vi "Get State from Child.vi"(8 "error in (no error)":errorcluster, 10 "Boolean":bool, 11 "Parent Actor in":refnum<class "Parent Actor.lvclass">) -> (0 "error out":errorcluster, 3 "Parent Actor out":refnum<class "Parent Actor.lvclass">)   [LabVIEW 2012, in "Parent Actor.lvclass"]
uses:
  Parent Actor.lvclass
  Parent Actor.lvclass/Parent Actor.ctl
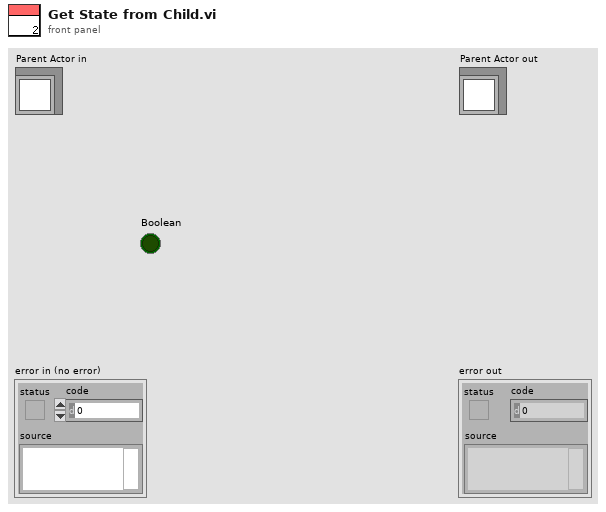
[diagram p1: front panel]
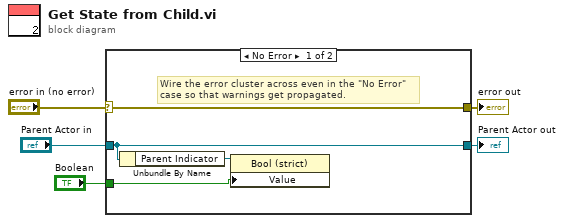
[diagram p0: block diagram]
diagram:
  n1 = case shown="No Error" "error in (no error)" {
    selector: "error in (no error)" -> [w9 w11]
    tunnel: [w9 w11] -> w4
    tunnel: [w8 w10] -> w2
    tunnel: "Parent Actor in" -> [w8 w10]
    tunnel: "Boolean" -> [w6 _]
    frame No Error {
      # "Wire the error cluster across even in the \"No Error\"\ncase so that warnings get propagated."
      n2 = Unbundle By Name(w8) -> ("Parent Indicator"=w7:refnum<vi>)
      n3 = property class="Bool (strict)"(reference=w7, "Value"=w6) -> ()  [unwired: 1 in, 2 out]
    }
    frame Error {
    }
  }
  "error out" <- w4
  "Parent Actor out" <- w2
